vi "Is First.vi"(8 "error in (no error)":errorcluster, 11 "Module ID":i32=-1) -> (0 "error out":errorcluster, 3 "First?":bool)   [LabVIEW 2020, in "FCR100.lvlib" / "Clone Registration.lvlib"]
doc: "Determine if the specified cloneable module ID was the first instance created.\n_____\nBased on DQMH Project Template 6.1.0.94."
uses:
  Clone Registration.lvlib
  Action--enum.ctl
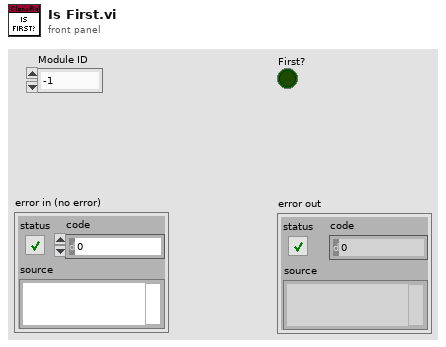
[diagram p1: front panel]
types:
  T1 = typedef "FCR100.lvlib/Clone Registration.lvlib/Action--enum.ctl" = enum16{"Init", "Add Instance", "Remove Instance", "List Instances", "Is First?"}
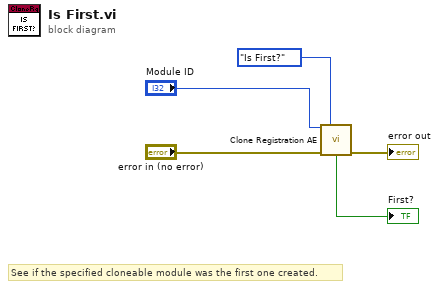
[diagram p0: block diagram]
diagram:
  # "See if the specified cloneable module was the first one created."
  n1 = call "Clone Registration AE.vi"("Module ID"="Module ID", "Action"=Action--enum."Is First?", "error in"="error in (no error)") -> ("First?"=→"First?":bool, "error out"=→"error out":errorcluster)  [unwired: 4 in, 7 out]
